vi "hdf5(SubVI).vi"(0 "Refnum in":refnum<k21>, 1 "VISA Refnum in":refnum<visa-resource-name>="GPIB0::19::INSTR", 2 "appended path":path, 3 "Max Voltage":dbl, 4 "error out 3":errorcluster, 5 "f":i32, 6 "SampClk.Rate":dbl, 7 "error in (no error)":errorcluster, 9 "drive_amplitude":dbl, 10 "task in":refnum<k21>, 13 "drive_freq":dbl, 17 "volt_div":dbl) -> (14 "task out 4":refnum<k21>, 16 "Array":dbl[][](array[numeric]), 18 "CC read error":errorcluster={"status"=FALSE, "code"=1073676294, "source"="VISA Read in datataker.vi"}, 20 "Refnum out":refnum<k21>, 21 "error out":errorcluster, 22 "error out 4":errorcluster, 23 "error out 2":errorcluster, 24 "Pirani pressure (mbar)":string, 25 "CC pressure (mbar)":string="2.4e", 26 "Temps (C):":dbl[](array[numeric])=[20.9, 21.3], 27 "error out":errorcluster={"status"=FALSE, "code"=1073676294, "source"="VISA Read in datataker.vi"})   [LabVIEW 2014]
uses:
  <vilib>/addons/h5labview2/file/H5F.lvlib
  <vilib>/addons/h5labview2/file/H5Fmode.ctl
  <vilib>/addons/h5labview2/group/H5G.lvlib
  <vilib>/addons/h5labview2/base/H5Equery.vi
  <vilib>/addons/h5labview2/base/lib_path.vi
  <vilib>/addons/h5labview2/dataset/H5Dwrite.llb/H5Dwrite.xnode
  <vilib>/addons/h5labview2/attrib/H5Awrite.llb/H5Awrite.xnode
  <vilib>/DAQmx/read.llb/DAQmx Read (Analog 2D DBL NChan NSamp).vi
  <vilib>/addons/h5labview2/base/hid_t.ctl
panel:
  out "Displacement":dbl format="%#.3f"
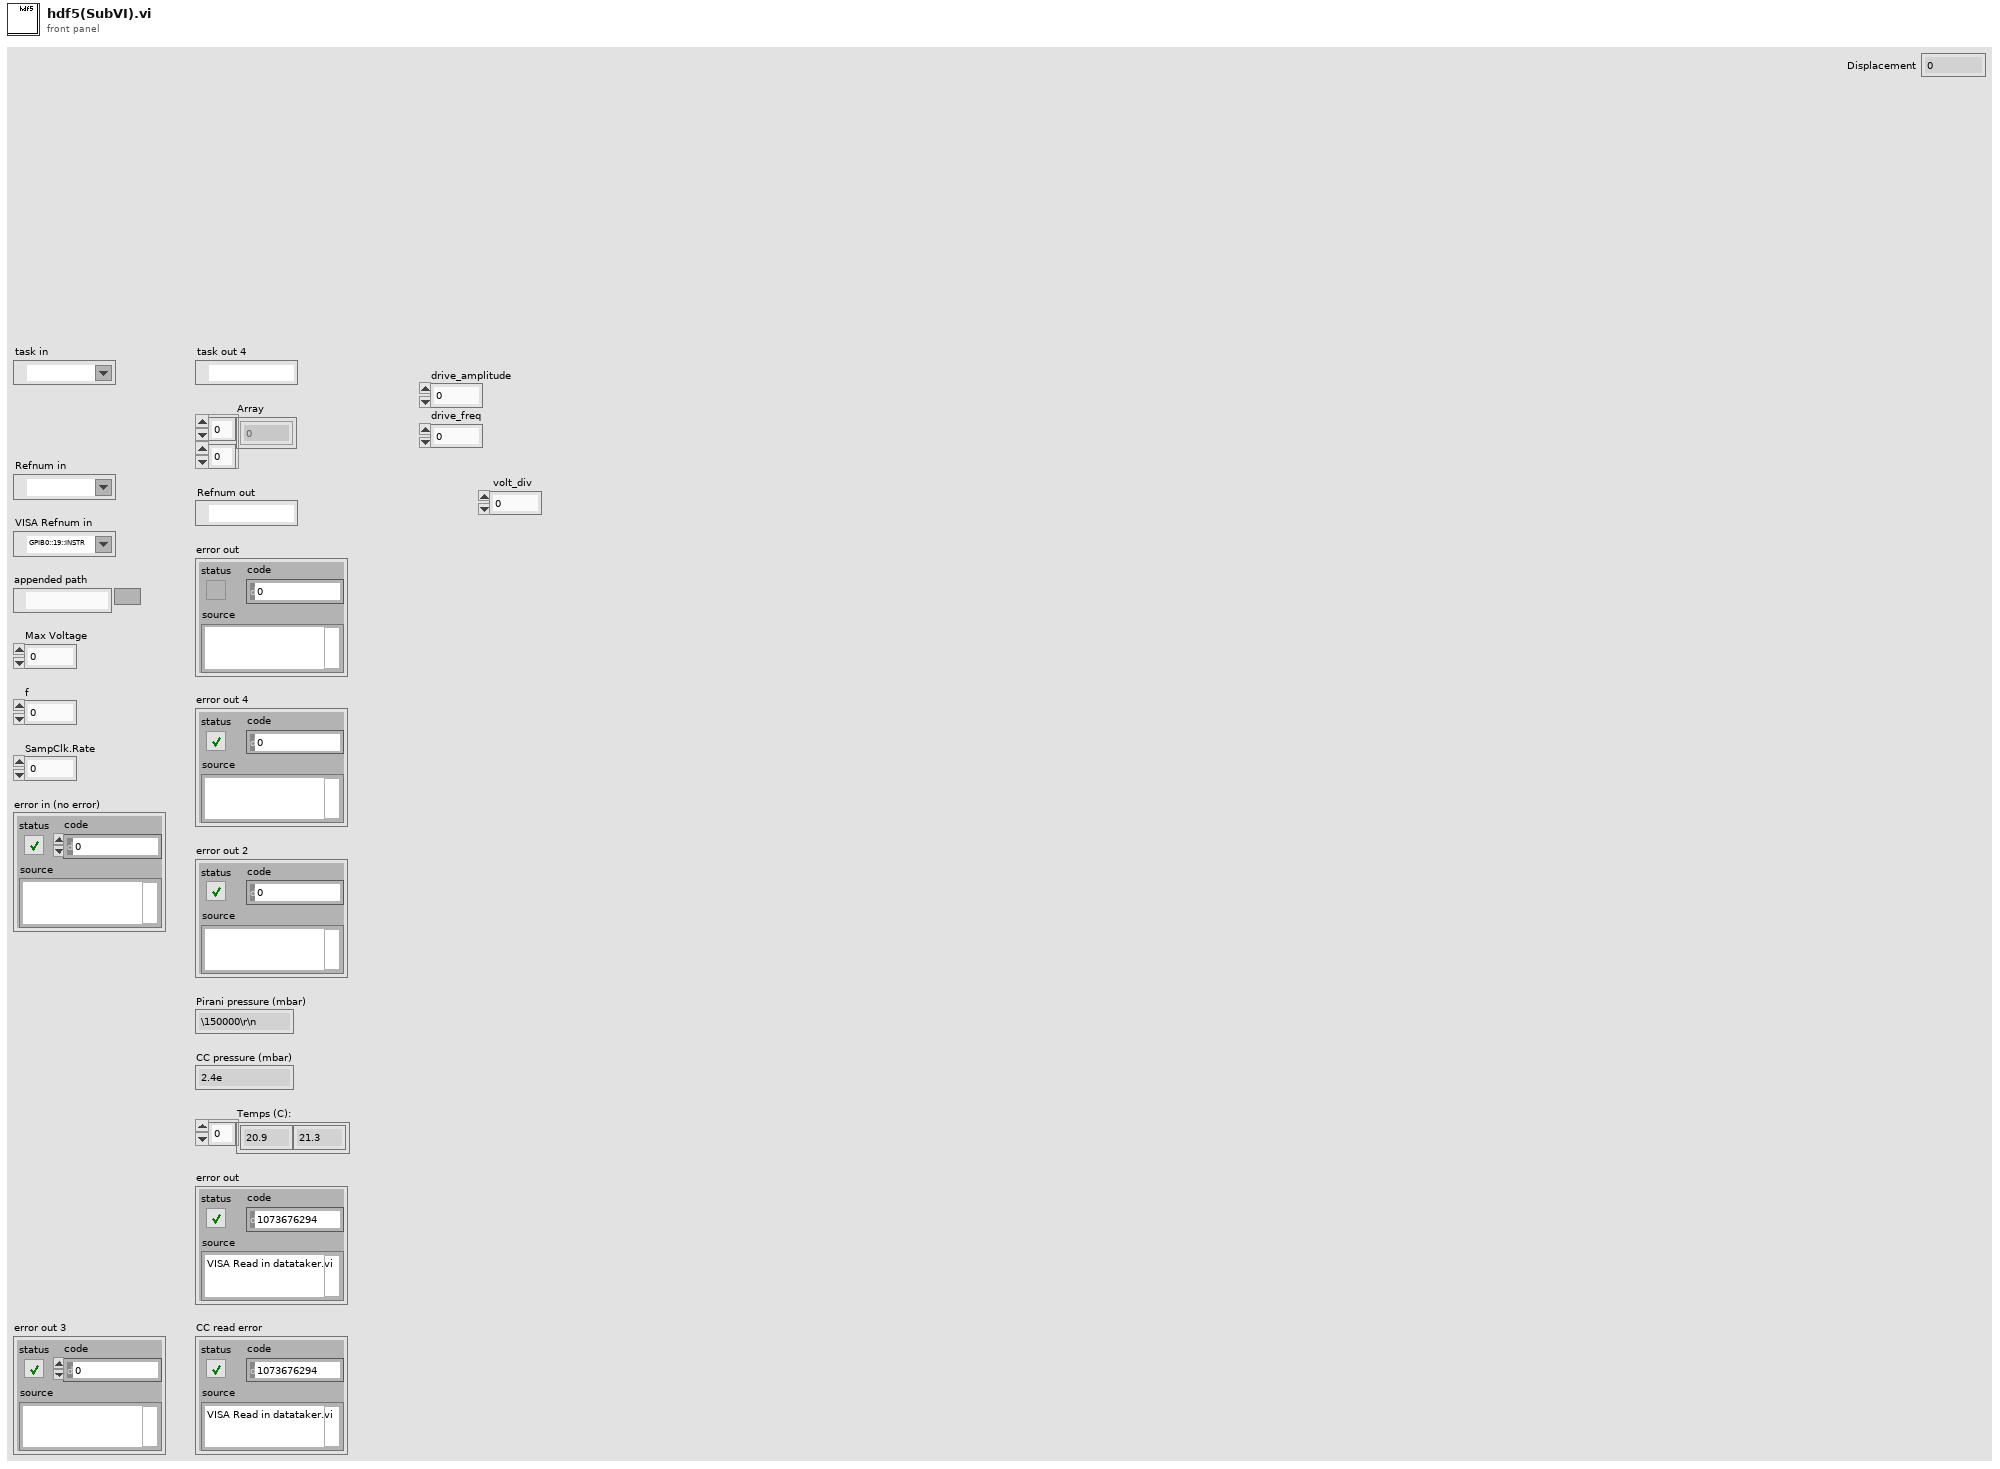
[diagram p1: front panel]
types:
  T1 = typedef "H5F.lvlib/H5Fmode.ctl" = enum16{"read-only", "read-write", "overwrite", "create new", "open or create"}
  T2 = typedef "hid_t.ctl" = i32
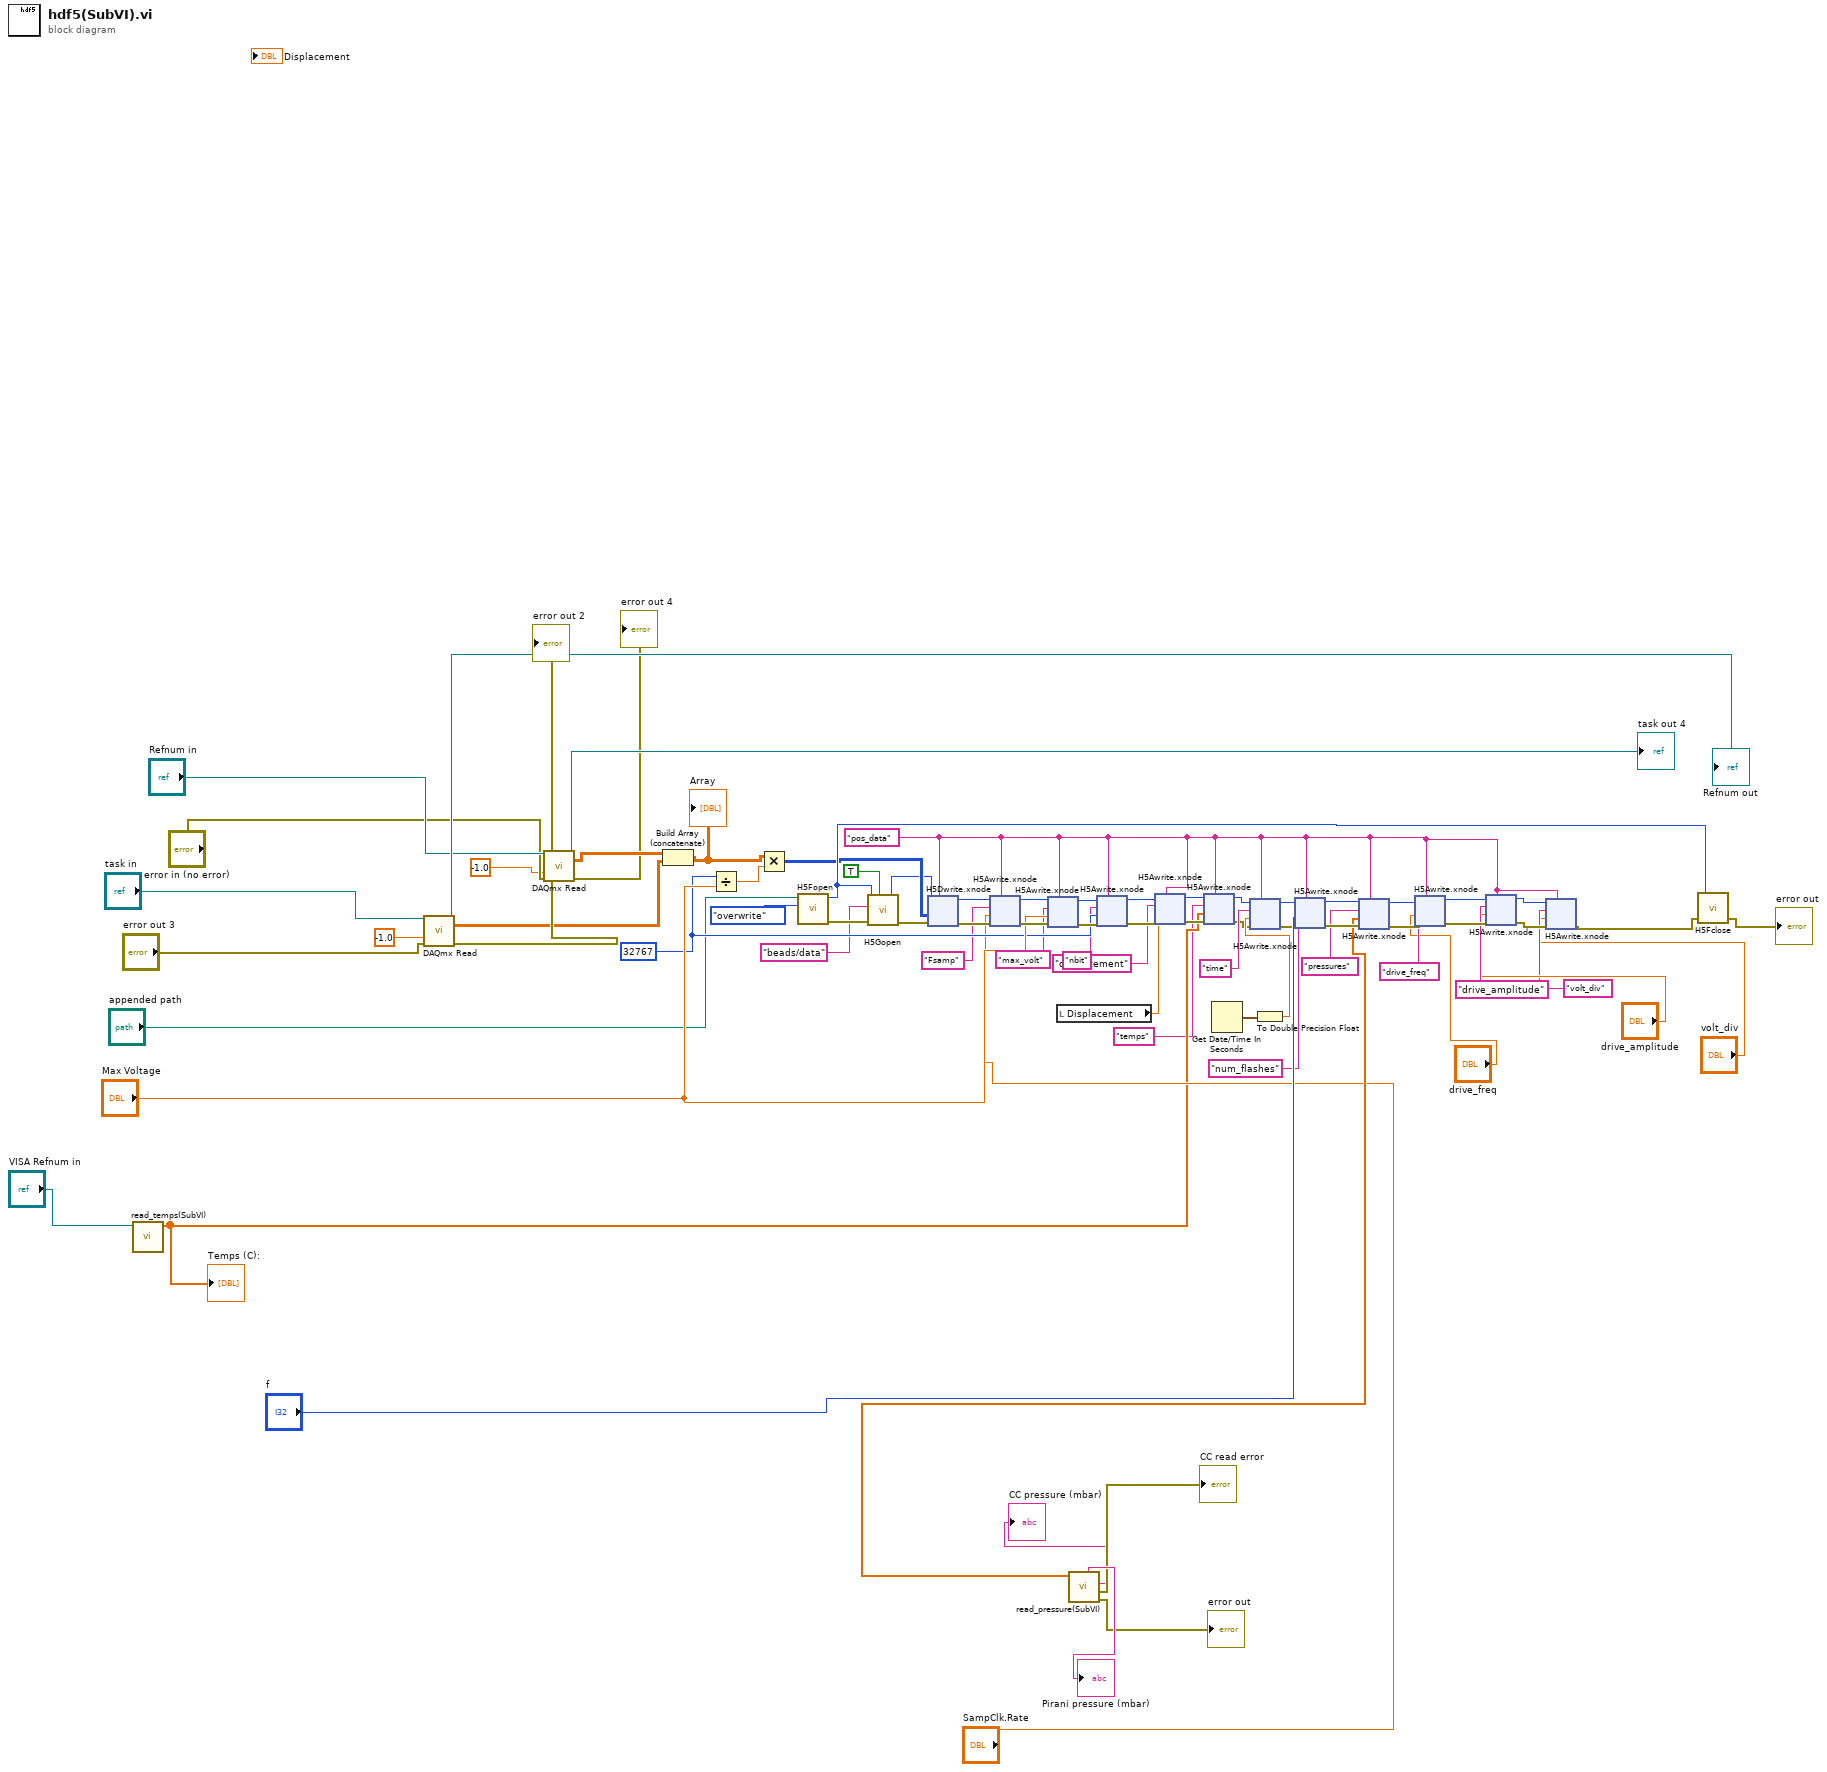
[diagram p0: block diagram]
diagram:
  w44 = i16 32767 ("y")
  w5 = "pos_data" ("dataset name")
  n1 = call "read_temps(SubVI).vi"("VISA Refnum in"="VISA Refnum in") -> ("Array"=w2:dbl[])  [unwired: 10 in]
  "Temps (C):" <- w2
  n2 = call-poly <vilib>:"DAQmx Read.vi"("task/channels in"="task in", "timeout"=-1.0, "error in"="error out 3") -> ("task out"=→"Refnum out":refnum<k21>, "data"=w63:dbl[][], "error out"=→"error out 2":errorcluster)  [unwired: 10 in]
  n3 = call-poly <vilib>:"DAQmx Read.vi"("task/channels in"="Refnum in", "timeout"=-1.0, "error in"="error in (no error)") -> ("task out"=→"task out 4":refnum<k21>, "data"=w62:dbl[][], "error out"=→"error out 4":errorcluster)  [unwired: 10 in]
  n4 = Build Array (concatenate)(w62, w63) -> (w64:dbl[][])
  "Array" <- w64
  n5 = Divide(x=w44, y="Max Voltage") -> (x/y=w43:dbl)
  n6 = Multiply(x=w64, y=w43) -> (x*y=w46:i16[][])
  n7 = call <vilib>:"H5Fopen.vi"("mode (read-only)"=H5Fmode."overwrite", "path"="appended path") -> ("error out"=w51:errorcluster, "ref out"=w56:T2)  [unwired: 4 in]
  n8 = call <vilib>:"H5Gopen.vi"("create? (F)"=TRUE, "error in (no error)"=w51, "name"="beads/data", "ref in"=w56) -> ("error out"=w52:errorcluster, "group out"=w30:T2)  [unwired: 3 in]
  n9 = xnode "H5Dwrite.xnode"("dataset name"=w5, "error in (no error)"=w52, "data"=w46, "ref in"=w30) -> ("error out"=w53:errorcluster, "ref out"=w31:i32)  [unwired: 3 in, 1 out]
  n10 = xnode "H5Awrite.xnode"("object name"=w5, "error in (no error)"=w53, "data"="SampClk.Rate", "attrib name"="Fsamp", "ref in"=w31) -> ("error out"=w54:errorcluster, "ref out"=w39:T2)  [unwired: 2 in, 1 out]
  n11 = xnode "H5Awrite.xnode"("object name"=w5, "error in (no error)"=w54, "data"="Max Voltage", "attrib name"="max_volt", "ref in"=w39) -> ("error out"=w55:errorcluster, "ref out"=w41:T2)  [unwired: 2 in, 1 out]
  n12 = local read "Displacement"() -> (w8:dbl)
  n13 = call "read_pressure(SubVI).vi"() -> ("error out"=→"error out":errorcluster, "CC read error"=→"CC read error":errorcluster, "CC pressure (mbar)"=→"CC pressure (mbar)":string, "Array"=w70:dbl[], "Pirani pressure (mbar)"=→"Pirani pressure (mbar)":string)  [unwired: 7 in]
  n14 = xnode "H5Awrite.xnode"("object name"=w5, "error in (no error)"=w55, "data"=w44, "attrib name"="nbit", "ref in"=w41) -> ("error out"=w10:errorcluster, "ref out"=w11:T2)  [unwired: 2 in, 1 out]
  n15 = xnode "H5Awrite.xnode"("object name"=w5, "error in (no error)"=w10, "data"=w8, "attrib name"="displacement", "ref in"=w11) -> ("error out"=w4:errorcluster, "ref out"=w7:T2)  [unwired: 2 in, 1 out]
  n16 = xnode "H5Awrite.xnode"("object name"=w5, "error in (no error)"=w4, "data"=w2, "attrib name"="temps", "ref in"=w7) -> ("error out"=w3:errorcluster, "ref out"=w6:T2)  [unwired: 2 in, 1 out]
  n17 = Get Date/Time In Seconds() -> (seconds since 1Jan1904=w49:timestamp)
  n18 = To Double Precision Float(number=w49) -> (double precision float=w50:dbl)
  n19 = xnode "H5Awrite.xnode"("object name"=w5, "error in (no error)"=w3, "data"=w50, "attrib name"="time", "ref in"=w6) -> ("error out"=w58:errorcluster, "ref out"=w57:T2)  [unwired: 2 in, 1 out]
  n20 = xnode "H5Awrite.xnode"("object name"=w5, "error in (no error)"=w58, "data"="f", "attrib name"="num_flashes", "ref in"=w57) -> ("error out"=w71:errorcluster, "ref out"=w69:T2)  [unwired: 2 in, 1 out]
  n21 = xnode "H5Awrite.xnode"("object name"=w5, "error in (no error)"=w71, "data"=w70, "attrib name"="pressures", "ref in"=w69) -> ("error out"=w25:errorcluster, "ref out"=w21:T2)  [unwired: 2 in, 1 out]
  n22 = xnode "H5Awrite.xnode"("object name"=w5, "error in (no error)"=w25, "data"="drive_freq", "attrib name"="drive_freq", "ref in"=w21) -> ("error out"=w24:errorcluster, "ref out"=w20:T2)  [unwired: 2 in, 1 out]
  n23 = xnode "H5Awrite.xnode"("object name"=w5, "error in (no error)"=w24, "data"="drive_amplitude", "attrib name"="drive_amplitude", "ref in"=w20) -> ("error out"=w16:errorcluster, "ref out"=w15:T2)  [unwired: 2 in, 1 out]
  n24 = xnode "H5Awrite.xnode"("object name"=w5, "error in (no error)"=w16, "data"="volt_div", "attrib name"="volt_div", "ref in"=w15) -> ("error out"=w14:errorcluster)  [unwired: 2 in, 2 out]
  n25 = call <vilib>:"H5Fclose.vi"("error in (no error)"=w14, "ref"=w56) -> ("error out"=→"error out":errorcluster)  [unwired: 3 in]
